vi "Within Tolerance.vi"(8 "tolerance":dbl, 10 "input":dbl, 11 "target":dbl) -> (3 "withinTolerance":bool)   [LabVIEW 2020]
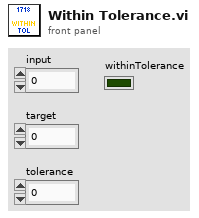
[diagram p1: front panel]
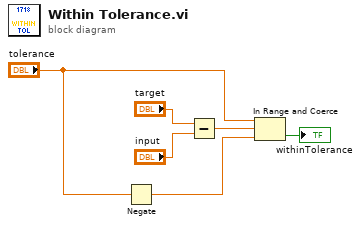
[diagram p0: block diagram]
diagram:
  n1 = Negate(x="tolerance") -> (-x=w3:dbl)
  n2 = Subtract(x="target", y="input") -> (x-y=w2:dbl)
  n3 = In Range and Coerce(upper limit="tolerance", x=w2, lower limit=w3) -> (In Range?=→"withinTolerance":bool)  [unwired: 1 out]
